vi "ws_log unsuccesful login.vi"(4 "session time (0.00)":dbl, 6 "username (\"\")":string, 8 "error in (no error)":errorcluster, 9 "Bad Bits (0)":u32, 10 "Log Bad Attempt? (f)":bool, 11 "Attempts (\"\")":i32) -> (0 "error out":errorcluster)   [LabVIEW 2011]
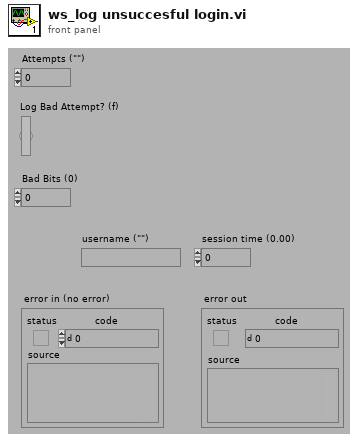
[diagram p1: front panel]
types:
  T1 = cluster{"Boolean array[0]":bool, "Boolean array[1]":bool, "Boolean array[2]":bool, "Boolean array[3]":bool}
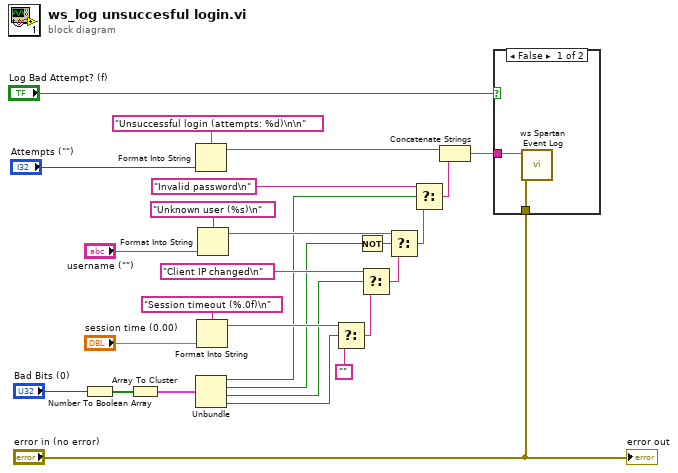
[diagram p0: block diagram]
diagram:
  n1 = Number To Boolean Array(number="Bad Bits (0)") -> (Boolean array=w6:bool[])
  n2 = Array To Cluster(array=w6) -> (cluster=w5:T1)
  n3 = Format Into String(format string="Unsuccessful login (attempts: %d)\n\n", "Attempts (\"\")") -> (resulting string=w19:string)  [unwired: 2 in, 1 out]
  n4 = Unbundle(w5) -> ("Boolean array[0]"=w4:bool, "Boolean array[1]"=w3:bool, "Boolean array[2]"=w2:bool, "Boolean array[3]"=w1:bool)
  n5 = Format Into String(format string="Session timeout (%.0f)\n", "session time (0.00)") -> (resulting string=w21:string)  [unwired: 2 in, 1 out]
  n6 = Format Into String(format string="Unknown user (%s)\n", "username (\"\")") -> (resulting string=w23:string)  [unwired: 2 in, 1 out]
  n7 = Select(t=w21, s=w1, f="") -> (s? t:f=w16:string)
  n8 = Not(x=w3) -> (.not. x?=w15:bool)
  n9 = Select(t="Client IP changed\n", s=w2, f=w16) -> (s? t:f=w17:string)
  n10 = Select(t=w23, s=w15, f=w17) -> (s? t:f=w20:string)
  n11 = Select(t="Invalid password\n", s=w4, f=w20) -> (s? t:f=w18:string)
  n12 = Concatenate Strings(w19, w18) -> (w14:string)
  n13 = case shown="False" "Log Bad Attempt? (f)" {
    tunnel: w14 -> [w29 _]
    tunnel: "error in (no error)" -> [w28 _]
    frame False {
      n14 = call "ws Spartan Event Log.vi"("error in (no error)"=w28, "message (\"\")"=w29) -> ()  [unwired: 6 in, 1 out]
    }
    frame True {
    }
  }
  "error out" <- "error in (no error)"
